vi "TEST - Variant Array to Spreadsheet.vi"(8 "error in (no error)":errorcluster) -> (0 "error out":errorcluster, 2 "pass":bool)   [LabVIEW 2020, in "test_openg_string.lvlib"]
uses:
  test_openg_string.lvlib
  <userlib>/_OpenG.lib/error/error.llb/openg_error.lvlib
  source/library/openg_string.lvlib
panel:
  out "Expected Result":string
  out "Result":string
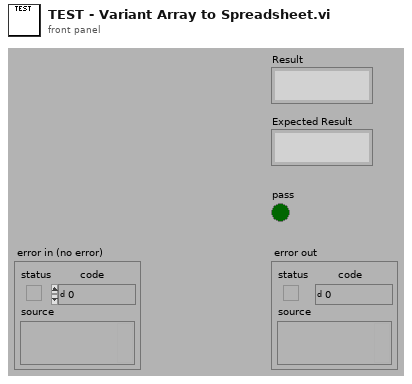
[diagram p1: front panel]
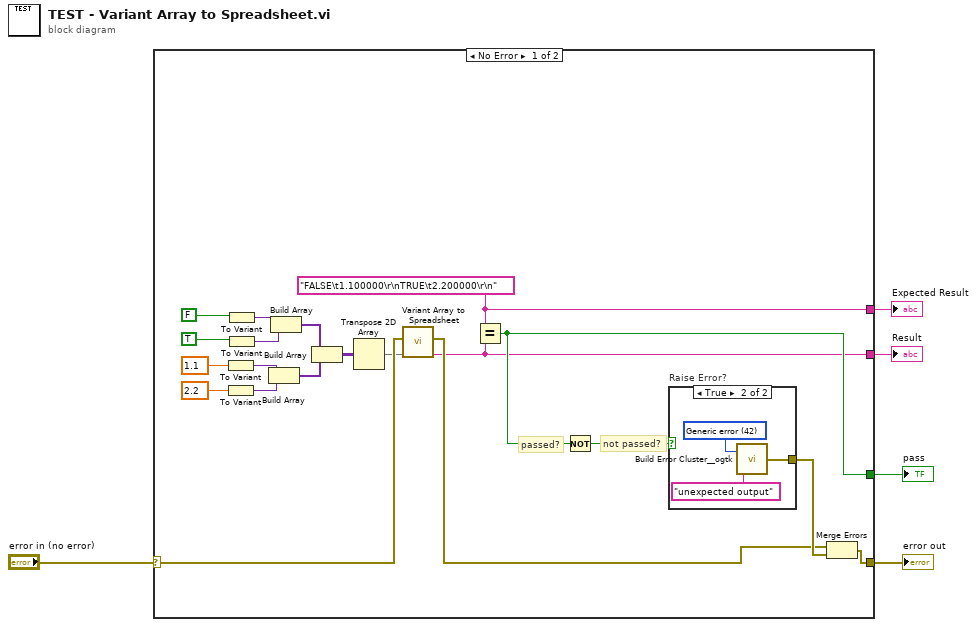
[diagram p0: block diagram]
diagram:
  n1 = case shown="No Error" "error in (no error)" {
    selector: "error in (no error)" -> [w9 w29]
    tunnel: [w22 _] -> w5
    tunnel: [w25 w29] -> w3
    tunnel: [w7 _] -> w2
    tunnel: [w6 _] -> w1
    frame No Error {
      w6 = "FALSE\t1.100000\r\nTRUE\t2.200000\r\n" ("Result")
      # "not passed?"
      # "passed?"
      n2 = To Variant(anything=1.1) -> (Variant=w15:variant)
      n3 = To Variant(anything=2.2) -> (Variant=w14:variant)
      n4 = To Variant(anything=FALSE) -> (Variant=w16:variant)
      n5 = To Variant(anything=TRUE) -> (Variant=w17:variant)
      n6 = Build Array(w15, w14) -> (w12:variant[])
      n7 = Build Array(w16, w17) -> (w13:variant[])
      n8 = Build Array(w13, w12) -> (w11:variant[][])
      n9 = Transpose 2D Array(2D array=w11) -> (transposed array=w8:variant[][])
      n10 = call "Variant Array to Spreadsheet.vi"("2D Variant Array"=w8, "error in (no error)"=w9) -> ("spreadsheet string"=w7:string, "error out"=w10:errorcluster)  [unwired: 8 in]
      n11 = Equal?(x=w6, y=w7) -> (x = y?=w22:bool)
      n12 = Not(x=w22) -> (.not. x?=w23:bool)
      n13 = case "Raise Error?" shown="True" w23 {
        tunnel: [_ w26] -> w24
        frame False {
        }
        frame True {
          w27 = 42 items=["No error", "Argument error", "Memory is full", "Out of zone", "End of file", "File already open", "Generic file I/O error", "File not found", "File permission error", "Disk is full", "Duplicate path", "Too many files open", "System feature not enabled", "Resource file not found", "Cannot add resource", "Resource not found", "Image not found", "Image memory error", "Pen does not exist", "Config type invalid", "Config token not found", "Config parse error", "Config memory error", "Bad external code format", "Bad external code offset", "External code not present", "Null window", "Destroy window error", "Null menu", "Print aborted", "Bad print record", "Print driver error", "Windows error during printing", "Memory error during printing", "Print dialog error", "Generic print error", "Invalid device refnum", "Device not found", "Device parameter error", "Device unit error", "Cannot open device", "Device call aborted", "Generic error", "Cancelled by user", "Object ID too low", "Object ID too high", "Object not in heap", "Unknown heap", "Unknown object (invalid DefProc)", "Unknown object (DefProc not in table)", "Message out of range", "Invalid (null) method", "Unknown message", "Manager call not supported", "Bad address", "Network operation in progress", "Network operation timed out", "Connection is busy", "Network attribute not supported", "Network error", "Address in use", "System out of memory", "Connection aborted", "Connection refused", "Not connected", "Already connected", "Connection closed", "Initialization error (interapplication manager)", "Bad occurrence", "Wait on unbound occurrence handler", "Occurrence queue overflow", "Datalog type conflict", "Unused", "Unrecognized type (interapplication manager)", "Memory corrupt", "Failed to make temporary DLL", "Old CIN version", "Drag socket not found", "Failed to load drop-object", "Failed to register OLE object", "Failed to release OLE object", "Format specifier type mismatch", "Unknown format specifier", "Too few format specifiers", "Too many format specifiers", "Scan failed", "Newer CIN version", "Error converting to variant", "Runtime menu error", "Password tampered", "Variant attribute not found", "Incompatible variant data type", "Event data is not available", "Event Store is not present", "Occurrence is not found", "Event Queue is not created", "Event info is not available", "Refnum passed is NULL", "Error retrieving Class GUID", "Error retrieving CoClass GUID", "Error retrieving TypeLib GUID.", "Bad built application magic bytes.", "Specific driver is different from the specific driver associated with the Logical Name.", "There is no session opened to the class driver.", "Max Error", "MAX - Error with config objects", "MAX - Error loading configuration", "MAX - Group not supported"]
          n14 = call <userlib>:"Build Error Cluster__ogtk.vi"("String to Prepend to source (\"\")"="unexpected output" ("String to Prepend to source (\"\")"), "code"=w27) -> ("error out"=w26:errorcluster)
        }
      }
      n15 = Merge Errors(w10, w24) -> (w25:errorcluster)
    }
    frame Error {
    }
  }
  "pass" <- w5
  "error out" <- w3
  "Result" <- w2
  "Expected Result" <- w1
